vi "Multiplexer Set Channel.vi"(8 "error in (no error)":errorcluster, 11 "Hardware Resources in":T1={"AIDAQ"="", "Signal Type"=enum."Sine Wave", "DODAQ"=""}) -> (0 "error out":errorcluster, 2 "Graph Data":waveform(dbl)[](array[waveform]), 3 "Hardware Resources out":T1={"AIDAQ"="", "Signal Type"=enum."Sine Wave", "DODAQ"=""})   [LabVIEW 2023, in "Acquisition.lvlib"]
doc: "Generates sample waveforms according to the signal type in the HW Config input."
uses:
  Acquisition.lvlib
  Hardware Configuration.ctl
  Signal Type.ctl
  <vilib>/DAQmx/read.llb/DAQmx Read (Analog 1D Wfm NChan 1Samp).vi
  <vilib>/DAQmx/write.llb/DAQmx Write (Digital 1D U8 1Chan NSamp).vi
  <vilib>/DAQmx/miscellaneous.llb/DAQmx Fill In Error Info.vi
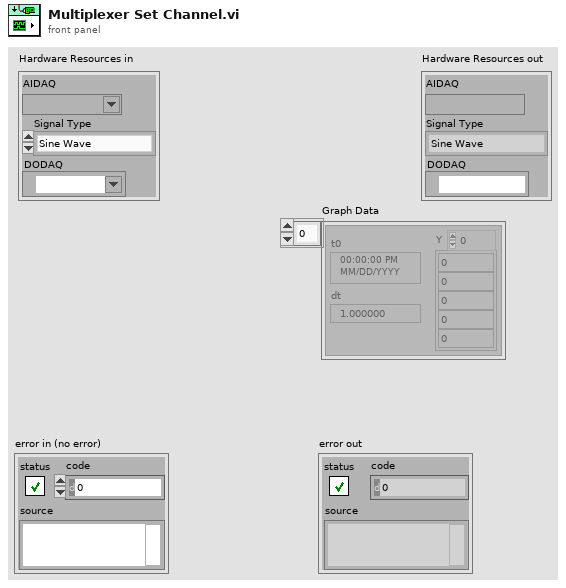
[diagram p1: front panel]
types:
  T1 = typedef "Acquisition.lvlib/Hardware Configuration.ctl" = cluster{"AIDAQ":refnum<k21>, "Signal Type":T2, "DODAQ":refnum<k21>}
  T2 = typedef "Acquisition.lvlib/Signal Type.ctl" = enum16{"cDAQ Thermistor", "cDAQ TC", "cDAQ RTD", "myDAQ Temp", "Sine Wave", "Square with Noise"}
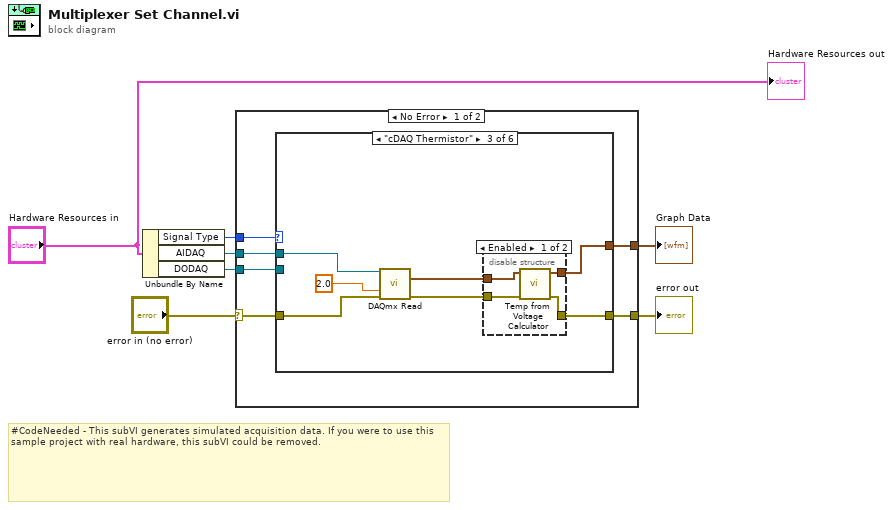
[diagram p0: block diagram]
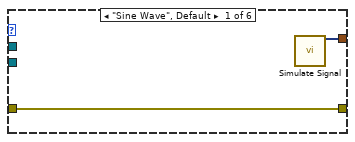
[diagram p2: hidden frame]
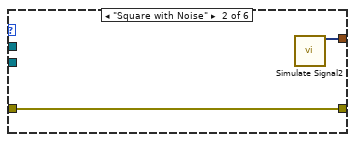
[diagram p3: hidden frame]
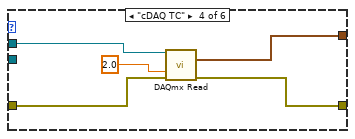
[diagram p5: hidden frame]
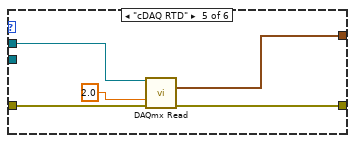
[diagram p6: hidden frame]
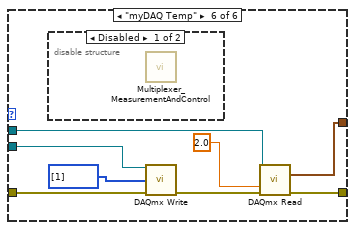
[diagram p7: hidden frame]
diagram:
  # "#CodeNeeded - This subVI generates simulated acquisition data. If you were to use this sample project with real hardware, this subVI could be removed."
  n1 = Unbundle By Name("Hardware Resources in") -> ("Signal Type"=w6:T2, "AIDAQ"=w4:refnum<k21>, "DODAQ"=w2:refnum<k21>)
  n2 = case shown="No Error" "error in (no error)" {
    selector: "error in (no error)" -> [w12 w49]
    tunnel: [w11 w49] -> w1
    tunnel: w6 -> [w13 _]
    tunnel: w4 -> [w10 _]
    tunnel: [w9 _] -> w3
    tunnel: w2 -> [w8 _]
    frame No Error {
      n3 = case shown="\"cDAQ Thermistor\"" w13 {
        tunnel: [w15 w17 w21 w33 w38 w45] -> w9
        tunnel: w12 -> [w14 w16 w24 w35 w39 w48]
        tunnel: [w14 w16 w18 w31 w36 w41] -> w11
        tunnel: w10 -> [_ _ w22 w32 w40 w43]
        tunnel: w8 -> [_ _ _ _ _ w42]
        frame "Sine Wave", Default {
          n4 = call "Simulate Signal"() -> ("Sine"=w15:dynamicdata)  [unwired: 14 in, 1 out]
        }
        frame "Square with Noise" {
          n5 = call "Simulate Signal2"() -> ("Square with Gaussian Noise"=w17:dynamicdata)  [unwired: 14 in, 1 out]
        }
        frame "cDAQ Thermistor" {
          n6 = call-poly <vilib>:"DAQmx Read.vi"("task/channels in"=w22, "timeout"=2.0, "error in"=w24) -> ("data"=w20:waveform(dbl)[], "error out"=w19:errorcluster)  [unwired: 10 in, 1 out]
          n7 = disable-structure shown="Enabled" {
            disable-tunnel: [w28 w30] -> w21
            disable-tunnel: w20 -> [w27 w30]
            disable-tunnel: w19 -> [w26 w29]
            disable-tunnel: [w25 w29] -> w18
            frame Enabled {
              n8 = call "Temp from Voltage Calculator.vi"("error in (no error)"=w26, "Graph Data 3"=w27) -> ("error out"=w25:errorcluster, "Graph Data 2"=w28:waveform(dbl)[])  [unwired: 7 in]
            }
            frame Disabled {
            }
          }
        }
        frame "cDAQ TC" {
          n9 = call-poly <vilib>:"DAQmx Read.vi"("task/channels in"=w32, "timeout"=2.0, "error in"=w35) -> ("data"=w33:waveform(dbl)[], "error out"=w31:errorcluster)  [unwired: 10 in, 1 out]
        }
        frame "cDAQ RTD" {
          n10 = call-poly <vilib>:"DAQmx Read.vi"("task/channels in"=w40, "timeout"=2.0, "error in"=w39) -> ("data"=w38:waveform(dbl)[], "error out"=w36:errorcluster)  [unwired: 10 in, 1 out]
        }
        frame "myDAQ Temp" {
          n11 = disable-structure shown="Disabled" {
            frame Disabled {
              n12 = call "Multiplexer_MeasurementAndControl.vi"() -> ()  [unwired: 9 in, 3 out]
            }
            frame Enabled {
            }
          }
          n13 = call-poly <vilib>:"DAQmx Write.vi"("task/channels in"=w42, "data"=u8[] [1], "error in"=w48) -> ("error out"=w46:errorcluster)  [unwired: 10 in, 2 out]
          n14 = call-poly <vilib>:"DAQmx Read.vi"("task/channels in"=w43, "timeout"=2.0, "error in"=w46) -> ("data"=w45:waveform(dbl)[], "error out"=w41:errorcluster)  [unwired: 10 in, 1 out]
        }
      }
    }
    frame Error {
    }
  }
  "error out" <- w1
  "Graph Data" <- w3
  "Hardware Resources out" <- "Hardware Resources in"
